vi "XDataNode12_0To11_0.vi"(10 "Version-State Cluster In":T1, 11 "XRef":refnum<vi>) -> (0 "Custom Label":string, 1 "Custom Warning To Issue":string, 2 "Version-State Cluster Out":T1, 3 "Action":T2)   [LabVIEW 2020]
uses:
  <vilib>/XSFPSupport/SFPChangeStateAction.ctl
  <vilib>/XNodeSupport/XNodeVersion.ctl
  <vilib>/XNodeSupport/XNodeUShort.ctl
  <vilib>/Platform/TimedLoop/XDataNode/XDataNode.ctl
  <vilib>/Platform/TimedLoop/XDataNode/timing_clust.ctl
  <vilib>/Platform/TimedLoop/XDataNode/nitl_modes.ctl
  <vilib>/Platform/TimedLoop/XDataNode/wakeup.ctl
  <vilib>/Platform/TimedLoop/XDataNode/TermInfo.ctl
  <vilib>/Platform/TimedLoop/XDataNode/nitl_TargetSpecificData.ctl
  <vilib>/Platform/TimedLoop/XDataNode/DN_Type.ctl
  <vilib>/XSFPSupport/NI_XSFPSupport.lvlib
  <vilib>/XNodeSupport/NI_XNodeSupport.lvlib
  <vilib>/Platform/TimedLoop/XDataNode/XDNodeRunTimeDep.lvlib
  <vilib>/Platform/TimedLoop/XDataNode/XDataNode.xnode
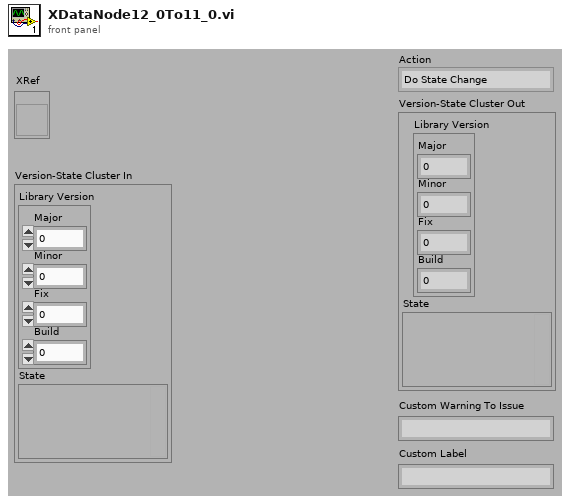
[diagram p1: front panel]
types:
  T1 = cluster{"Library Version":cluster{"Major":u16, "Minor":u16, "Fix":u16, "Build":u16}, "State":variant}
  T2 = typedef "NI_XSFPSupport.lvlib/SFPChangeStateAction.ctl" = enum32{"Do State Change", "Replace With Label", "Fail SFP"}
  T3 = typedef "NI_XNodeSupport.lvlib/XNodeVersion.ctl" = cluster{"Major":T4, "Minor":T4, "Fix":T4, "Build":T4}
  T4 = typedef "NI_XNodeSupport.lvlib/XNodeUShort.ctl" = u16
  T5 = cluster{"Major":u16, "Minor":u16, "Fix":u16, "Build":u16}
  T6 = typedef "XDataNode.xnode/nitl_TargetSpecificData.ctl" = cluster{"Target Name":string, "Target Data":variant}
  T7 = typedef "XDataNode.xnode/XDataNode.ctl" = cluster{"Timing":T8, "Size":T11[], "Hidden":T11[], "Invisible":bool[], "Input?":bool, "timing src wired?":bool, "Target Specific Data":T6[], "G Only Data":variant, "DataNode_Type":T12}
  T8 = typedef "XDNodeRunTimeDep.lvlib/timing_clust.ctl" = cluster{"Expected End [f-1]":u64, "Actual End [f-1]":u64, "Finished Late? [f-1]":bool, "Expected End [i-1]":u64, "Actual End [i-1]":u64, "Finished Late? [i-1]":bool, "Expected Start [i]":u64, "Actual Start [i]":u64, "Expected Start [f]":u64, "Actual Start [f]":u64, "Source Name":string, "Structure Name":string, "Period":i64, "Deadline":i64, "Offset":i64, "Start":i64, "Priority":i32, "Timeout":i32, "Mode":T9, "Wakeup Reason":T10, "Error":errorcluster, "Source Type":string, "Secondary Source Type":string, "Global End Time":u64, "Global Start Time":u64, "Frame Duration":u64, "Iteration Duration":u64, "Assigned CPU":i32, "I/O Scan Engine Mode":u32}
  T9 = typedef "XDNodeRunTimeDep.lvlib/nitl_modes.ctl" = enum32{"No Change", "Process missed periods, maintain original phase", "Discard missed periods, maintain original phase", "Process missed periods, ignore original phase", "Discard missed periods, ignore original phase"}
  T10 = typedef "XDNodeRunTimeDep.lvlib/wakeup.ctl" = enum32{"Normal", "Aborted", "Asynchronous wakeup", "Timing source error", "Timed loop error", "Timeout"}
  T11 = typedef "XDataNode.xnode/TermInfo.ctl" = cluster{"ID":i32, "Wired?":bool, "Type":variant, "Name":string, "Input?":bool, "StaticID":i32}
  T12 = typedef "XDataNode.xnode/DN_Type.ctl" = enum32{"TL_Lft_Ear", "TL_Rt_Ear", "TL_Lft_Dn", "TL_Rt_Dn", "TS_Lft_Ear", "TS_Rt_Ear", "TS_1stFrame_Lft_Dn", "TS_Lft_Dn", "TS_LastFrame_Rt_Dn", "TS_Rt_Dn", "TL_TS_Lft_Ear", "TL_TS_Rt_Ear", "TL_TS_Lft_Dn", "TL_TS_Rt_Dn", "TL_TS_1stFrame_Lft_Dn", "TL_TS_LastFrame_Rt_Dn"}
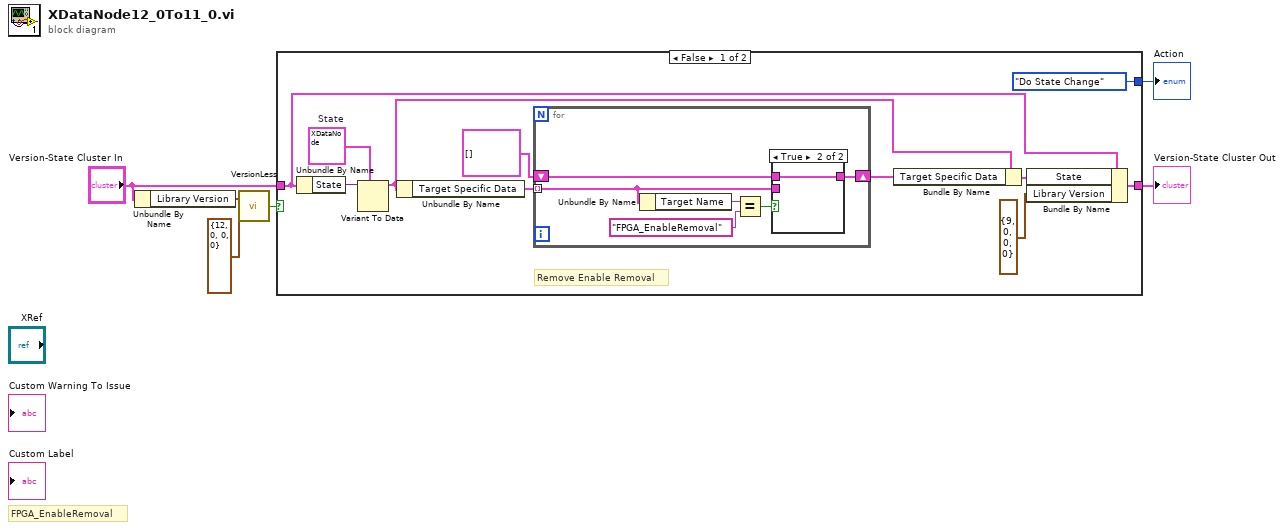
[diagram p0: block diagram]
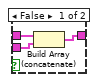
[diagram p2: hidden frame]
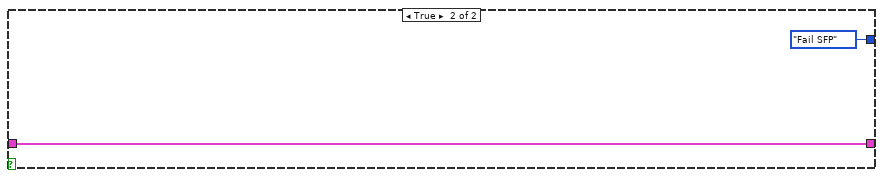
[diagram p3: hidden frame]
diagram:
  # "FPGA_EnableRemoval"
  n1 = Unbundle By Name("Version-State Cluster In") -> ("Library Version"=w3:T5)
  n2 = call <vilib>:"VersionLess.vi"("y"=T3 {"Major"=12, "Minor"=0, "Fix"=0, "Build"=0}, "x"=w3) -> ("x < y?"=w5:bool)
  n3 = case shown="False" w5 {
    tunnel: [SFPChangeStateAction."Do State Change" ("Action") SFPChangeStateAction."Fail SFP" ("Action")] -> w4
    tunnel: [w16 w28] -> w2
    tunnel: "Version-State Cluster In" -> [w13 w28]
    frame False {
      w14 = T7 {"Timing"={"Expected End [f-1]"=0, "Actual End [f-1]"=0, "Finished Late? [f-1]"=FALSE, "Expected End [i-1]"=0, "Actual End [i-1]"=0, "Finished Late? [i-1]"=FALSE, "Expected Start [i]"=0, "Actual Start [i]"=0, "Expected Start [f]"=0, "Actual Start [f]"=0, "Source Name"="", "Structure Name"="", "Period"=0, "Deadline"=0, "Offset"=0, "Start"=0, "Priority"=0, "Timeout"=0, "Mode"=enum."No Change", "Wakeup Reason"=enum."Normal", "Error"={"status"=FALSE, "code"=0, "source"=""}, "Source Type"="", "Secondary Source Type"="", "Global End Time"=0, "Global Start Time"=0, "Frame Duration"=0, "Iteration Duration"=0, "Assigned CPU"=0, "I/O Scan Engine Mode"=0}, "Size"=[], "Hidden"=[], "Invisible"=[], "Input?"=FALSE, "timing src wired?"=FALSE, "Target Specific Data"=[], "G Only Data"=variant, "DataNode_Type"=enum."TL_Lft_Ear"}  # State
      # "Remove Enable Removal"
      n4 = Unbundle By Name(w13) -> ("State"=w12:variant)
      n5 = Variant To Data(type=w14, Variant=w12) -> (data=w9:T7)  [unwired: 1 in, 1 out]
      n6 = Unbundle By Name(w9) -> ("Target Specific Data"=w11:T6[])
      n7 = for {
        tunnel: w11 -> [w20] mode=indexing
        shift-right: [w18] -> w8
        shift-left: T6[] [] ("Target Specific Data") -> [w19]
        n8 = Unbundle By Name(w20) -> ("Target Name"=w23:string)
        n9 = Equal?(x=w23, y="FPGA_EnableRemoval" ("Target Name")) -> (x = y?=w21:bool)
        n10 = case shown="True" w21 {
          tunnel: w20 -> [w26 _]
          tunnel: w19 -> [w25 w27]
          tunnel: [w24 w27] -> w18
          frame False {
            n11 = Build Array (concatenate)(w25, w26) -> (w24:T6[])
          }
          frame True {
          }
        }
      }
      n12 = Bundle By Name(cluster=w9, "Target Specific Data"=w8) -> (w7:T7)
      n13 = Bundle By Name(cluster=w13, "State"=w7, "Library Version"=T3 {"Major"=9, "Minor"=0, "Fix"=0, "Build"=0} ("y")) -> (w16:T1)
    }
    frame True {
    }
  }
  "Action" <- w4
  "Version-State Cluster Out" <- w2
